vi "NHMFL-LSCI234 In-Out.vi"(2 "Port Number":T1=65535 items=["Modem", "Printer", "COM3", "COM4", "COM5", "COM6", "COM7", "COM8", "COM9", "Nothing", "LPT1", "LPT2", "LPT3", "LPT4"], 3 "Comand String":string="OHMS?\r\n") -> (0 "Return Value":dbl=108.958 format="%.3f", 1 "Return String":string="108.958\r\n")   [LabVIEW 2024]
uses:
  Serial Instruments/Serial Support VISA.llb/Communication Port.ctl
  Serial Instruments/Serial Support VISA.llb/Serial Actions.ctl
panel:
  out "?":bool
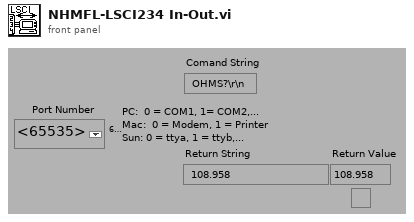
[diagram p1: front panel]
types:
  T1 = typedef "Communication Port.ctl" = u16
  T2 = typedef "Serial Actions.ctl" = enum16{"Init", "Break", "Clear Buffer", "Write", "Read", "N Bytes", "Lock", "Unlock", "Close"}
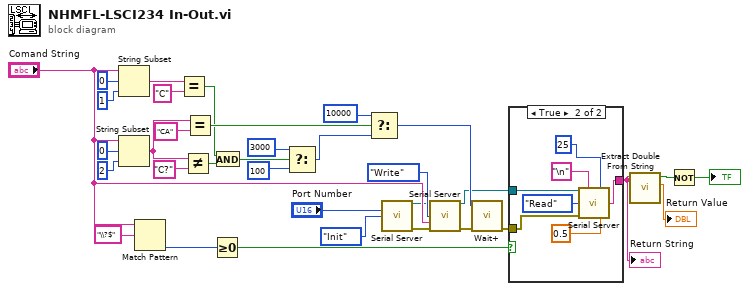
[diagram p0: block diagram]
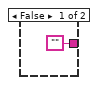
[diagram p2: hidden frame]
diagram:
  n1 = String Subset(string="Comand String", offset (0)=0, length (rest)=1) -> (substring=w15:string)
  n2 = String Subset(string="Comand String", offset (0)=0, length (rest)=2) -> (substring=w22:string)
  n3 = Match Pattern(string="Comand String", regular expression="\\?$") -> (offset past match=w10:i32)  [unwired: 1 in, 3 out]
  n4 = Equal?(x=w15, y="C") -> (x = y?=w19:bool)
  n5 = Not Equal?(x=w22, y="C?") -> (x != y?=w20:bool)
  n6 = Equal?(x=w22, y="CA") -> (x = y?=w25:bool)
  n7 = Greater Or Equal To 0?(x=w10) -> (x >= 0?=w11:bool)
  n8 = And(x=w19, y=w20) -> (x .and. y?=w21:bool)
  n9 = Select(t=u32 3000, s=w21, f=u32 100) -> (s? t:f=w26:u32)
  n10 = Select(t=u32 10000, s=w25, f=w26) -> (s? t:f=w3:u32)
  n11 = call "Serial Server.vi"("Port Number"="Port Number", "Action"=Serial_Actions."Init") -> ("dup VISA Resource Name"=w6:refnum<visa-resource-name>, "error out"=w29:errorcluster)  [unwired: 9 in, 3 out]
  n12 = call "Serial Server.vi"("VISA Resource Name"=w6, "Action"=Serial_Actions."Write", "String To Send"="Comand String", "error in (no error)"=w29) -> ("dup VISA Resource Name"=w1:refnum<visa-resource-name>, "error out"=w5:errorcluster)  [unwired: 7 in, 3 out]
  n13 = call "Wait+.vi"("Error In"=w5, "milliseconds to wait"=w3) -> ("Error Out"=w4:errorcluster)  [unwired: 4 in, 1 out]
  n14 = case shown="True" w11 {
    tunnel: ["" w41] -> w8
    tunnel: w4 -> [_ w39]
    tunnel: w1 -> [_ w36]
    frame False {
    }
    frame True {
      n15 = call "Serial Server.vi"("VISA Resource Name"=w36, "EOT Chars (cr/lf)"="\n", "Max Char to Read"=25, "Action"=Serial_Actions."Read", "error in (no error)"=w39, "Timeout Limit(sec)"=0.5) -> ("Serial Read"=w41:string)  [unwired: 5 in, 4 out]
    }
  }
  "Return String" <- w8
  n16 = call "Extract Double From String.vi"("string"=w8) -> ("floating pt. number"=→"Return Value":dbl, "valid"=w33:bool)  [unwired: 3 in, 2 out]
  n17 = Not(x=w33) -> (.not. x?=→"?":bool)
